vi "Write Measurment.vi"() -> ()   [LabVIEW 2022 SP3]
uses:
  <vilib>/measure/NI_MABase.lvlib
panel:
  out "Waveform Chart":waveform(dbl)(graph)
  in  "Amplitude":dbl(knob) scale=0.0..10.0
  in  "Frequency":dbl(knob) scale=0.0..10.0
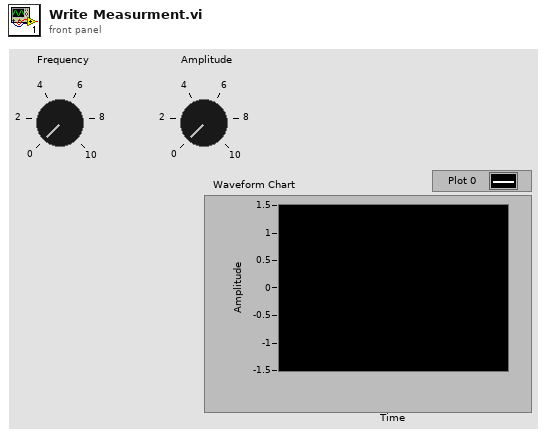
[diagram p1: front panel]
types:
  T1 = enum16{"Sine Wave", "Triangle Wave", "Square Wave", "Sawtooth Wave"}
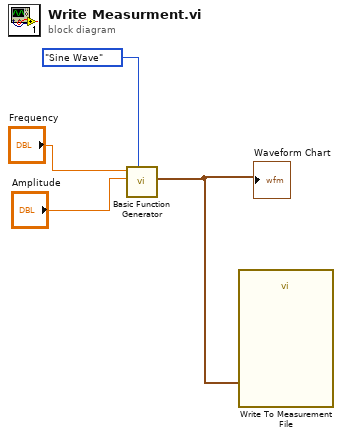
[diagram p0: block diagram]
diagram:
  n1 = call <vilib>:"Basic Function Generator.vi"("signal type"=T1."Sine Wave", "amplitude"="Amplitude", "frequency"="Frequency") -> ("signal out"=w1:waveform(dbl))  [unwired: 6 in, 2 out]
  "Waveform Chart" <- w1
  n2 = call "Write To Measurement File"("Signals"=w1) -> ()  [unwired: 16 in, 3 out]
